vi "Read Voltage.vi"(8 "error in (no error)":errorcluster, 11 "AIO in":refnum<class "AIO.lvclass">) -> (0 "error out":errorcluster, 2 "Status":string, 3 "AIO out":refnum<class "AIO.lvclass">)   [LabVIEW 2020, in "AIO.lvclass"]
uses:
  AIO.lvclass
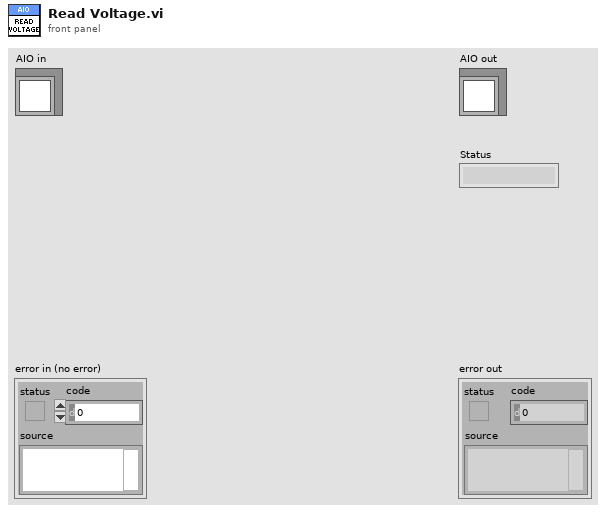
[diagram p1: front panel]
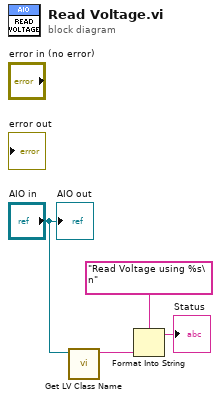
[diagram p0: block diagram]
diagram:
  n1 = call <vilib>:"Get LV Class Name.vi"("object"="AIO in") -> ("class name"=w4:string)  [unwired: 9 in, 1 out]
  n2 = Format Into String(format string="Read Voltage using %s\n", w4) -> (resulting string=→"Status":string)  [unwired: 2 in, 1 out]
  "AIO out" <- "AIO in"
